vi "Start Multisampling and Wait for Finish.vi"(5 "status string ref.":refnum<vi>, 6 "time resolution (0.1 s)":dbl=0.1, 7 "stop button ref.":refnum<vi>, 8 "error in":errorcluster, 10 "timeout":dbl, 11 "instrument handles":refnum<k15>[](array[refnum])) -> (0 "error out":errorcluster, 2 "timeout exceeded?":bool, 3 "instrument handles out":refnum<k15>[](array[refnum]))   [LabVIEW 2013, in "varilib.lvlib"]
doc: "Starts sampling of NI SCOPE digitizers, and wait till sampling finished, or timeout was exceeded, or stop button was pressed. Stop button is optional. If reference of string control is wired, a status message with time left till timeout is generated. The time resolution sets the speed of loop, updating of status message or reading of stop button value.\nIf one of digitizers is master, it should be a first element in \"instrument handles\" array and it will be initiated as last one."
uses:
  varilib.lvlib
  <vilib>/Utility/error.llb/Error Cluster From Error Code.vi
  <vilib>/ErrorRing/Error Ring.xnode
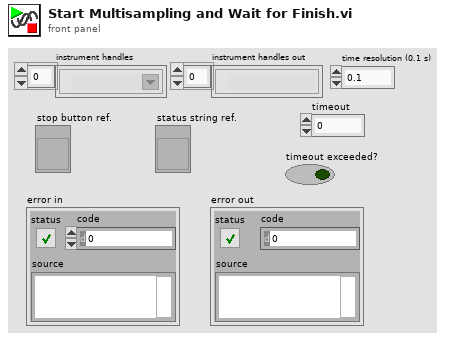
[diagram p1: front panel]
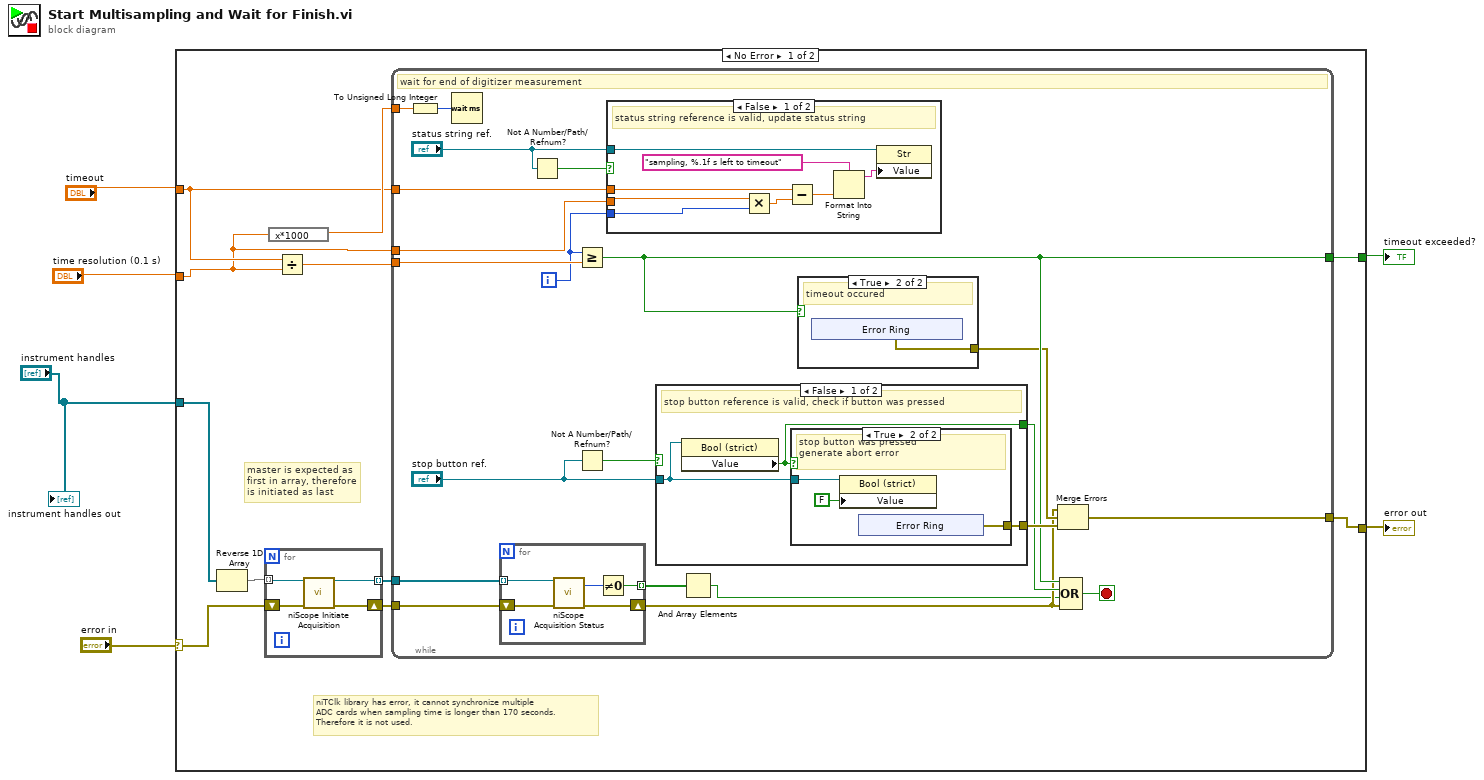
[diagram p0: block diagram]
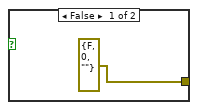
[diagram p2: hidden frame]
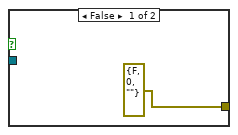
[diagram p3: hidden frame]
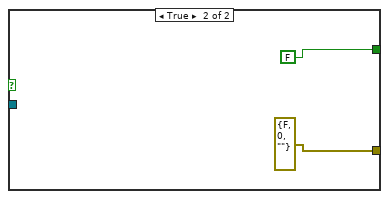
[diagram p4: hidden frame]
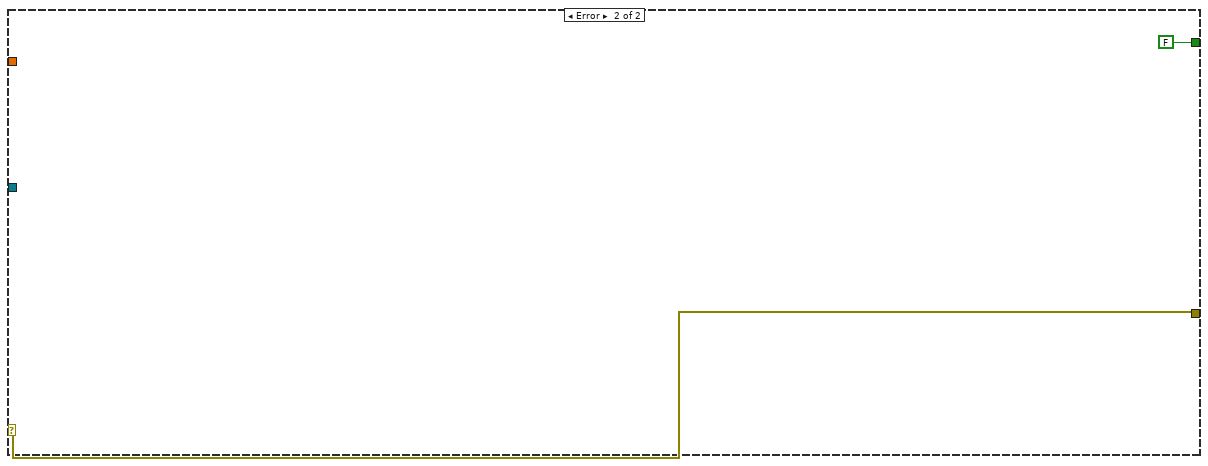
[diagram p6: hidden frame]
diagram:
  n1 = case shown="No Error" "error in" {
    selector: "error in" -> [w9 w78]
    tunnel: [w17 w78] -> w6
    tunnel: [w16 FALSE] -> w5
    tunnel: "timeout" -> [w13 _]
    tunnel: "time resolution (0.1 s)" -> [w12 _]
    tunnel: "instrument handles" -> [w11 _]
    frame No Error {
      # "master is expected as\nfirst in array, therefore\nis initiated as last"
      # "niTClk library has error, it cannot synchronize multiple\nADC cards when sampling time is longer than 170 seconds.\nTherefore it is not used."
      n2 = Reverse 1D Array(array=w11) -> (reversed array=w10:refnum<k15>[])
      n3 = for {
        tunnel: w10 -> [w21] mode=indexing
        shift-right: [w19] -> w8
        shift-left: w9 -> [w20]
        tunnel: [w18] -> w7 mode=indexing
        n4 = call <instrlib>:"niScope Initiate Acquisition.vi"("instrument handle"=w21, "error in"=w20) -> ("instrument handle out"=w18:refnum<k15>, "error out"=w19:errorcluster)  [unwired: 12 in]
      }
      n5 = expression code="x*1000"(w12) -> (w15:dbl)
      n6 = Divide(x=w13, y=w12) -> (x/y=w14:dbl)
      n7 = while {
        tunnel: w8 -> [w26]
        tunnel: [w41] -> w17
        tunnel: [w29] -> w16
        tunnel: w14 -> [w37]
        tunnel: w15 -> [w40]
        tunnel: w13 -> [w38]
        tunnel: w12 -> [w35]
        tunnel: w7 -> [w24]
        i -> [w36]
        stop <- w42 stop-if-true
        # "wait for end of digitizer measurement"
        n8 = To Unsigned Long Integer(number=w40) -> (unsigned 32bit integer=w39:u32)
        n9 = Wait (ms)(milliseconds to wait=w39) -> ()  [unwired: 1 out]
        n10 = for {
          tunnel: [w45] -> w23 mode=indexing
          tunnel: w24 -> [w44] mode=indexing
          shift-right: [w46] -> w25
          shift-left: w26 -> [w47]
          n11 = call <instrlib>:"niScope Acquisition Status.vi"("instrument handle"=w44, "error in"=w47) -> ("acquisition status"=w43:i32, "error out"=w46:errorcluster)  [unwired: 11 in, 1 out]
          n12 = Not Equal To 0?(x=w43) -> (x != 0?=w45:bool)
        }
        n13 = Not A Number/Path/Refnum?(number/path/refnum="status string ref.") -> (NaN/Path/Refnum?=w32:bool)
        n14 = Greater Or Equal?(x=w36, y=w37) -> (x >= y?=w29:bool)
        n15 = Not A Number/Path/Refnum?(number/path/refnum="stop button ref.") -> (NaN/Path/Refnum?=w30:bool)
        n16 = case shown="False" w32 {
          tunnel: w38 -> [w74 _]
          tunnel: w36 -> [w72 _]
          tunnel: w35 -> [w71 _]
          tunnel: "status string ref." -> [w69 _]
          frame False {
            # "status string reference is valid, update status string"
            n17 = Multiply(x=w71, y=w72) -> (x*y=w70:dbl)
            n18 = Subtract(x=w74, y=w70) -> (x-y=w73:dbl)
            n19 = Format Into String(format string="sampling, %.1f s left to timeout", w73) -> (resulting string=w75:string)  [unwired: 2 in, 1 out]
            n20 = property class="Str"(reference=w69, "Value"=w75) -> ()  [unwired: 1 in, 2 out]
          }
          frame True {
          }
        }
        n21 = case shown="False" w30 {
          tunnel: [w57 FALSE ("Value")] -> w27
          tunnel: [w56 errorcluster {"status"=FALSE, "code"=0, "source"=""} ("error out")] -> w34
          tunnel: "stop button ref." -> [w55 _]
          frame False {
            # "stop button reference is valid, check if button was pressed"
            n22 = property class="Bool (strict)"(reference=w55) -> ("Value"=w57:bool)  [unwired: 1 in, 2 out]
            n23 = case shown="True" w57 {
              tunnel: [errorcluster {"status"=FALSE, "code"=0, "source"=""} ("error out") w61] -> w56
              tunnel: w55 -> [_ w59]
              frame False {
              }
              frame True {
                # "stop button was pressed\ngenerate abort error"
                n24 = property class="Bool (strict)"(reference=w59, "Value"=FALSE) -> ()  [unwired: 1 in, 2 out]
                n25 = xnode "Error Ring"() -> ("error out"=w61:errorcluster)
              }
            }
          }
          frame True {
          }
        }
        n26 = And Array Elements(Boolean array=w23) -> (logical AND=w22:bool)
        n27 = case shown="True" w29 {
          tunnel: [errorcluster {"status"=FALSE, "code"=0, "source"=""} ("error out") w49] -> w28
          frame False {
          }
          frame True {
            # "timeout occured"
            n28 = xnode "Error Ring"() -> ("error out"=w49:errorcluster)
          }
        }
        n29 = Merge Errors(w25, w28, w34) -> (w41:errorcluster)
        n30 = Compound Arithmetic op=OR(w29, w27, w22, w25) -> (w42:bool)
      }
    }
    frame Error {
    }
  }
  "error out" <- w6
  "timeout exceeded?" <- w5
  "instrument handles out" <- "instrument handles"
